vi "DeviceSwitch.vi"(8 "error in (no error)":errorcluster caption="错误输入（无错误）", 9 "Device Index":i32, 10 "Open":bool, 11 "handle":u64) -> (0 "error out":errorcluster caption="错误输出", 2 "function return":i32, 3 "handle out":u64, 5 "Description":string, 7 "SerialNumber":string)   [LabVIEW 2018]
doc: "Set Open True to open device by Device Index or False to close device by handle."
uses:
  InstrumentsPlayground.lvlib
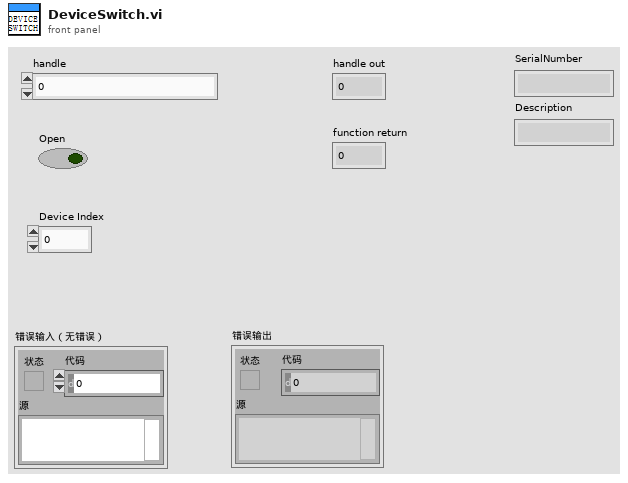
[diagram p1: front panel]
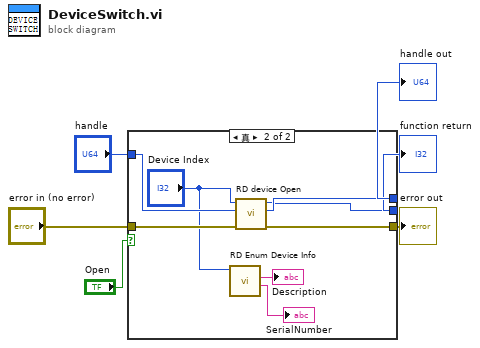
[diagram p0: block diagram]
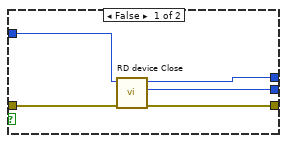
[diagram p2: hidden frame]
diagram:
  n1 = case shown="真" "Open" {
    tunnel: "handle" -> [w11 w18]
    tunnel: [w10 w16] -> w4
    tunnel: [w9 w15] -> w3
    tunnel: [w8 w19] -> w2
    tunnel: "error in (no error)" -> [w7 w17]
    frame False {
      n2 = call "RD device Close.vi"("error in (no error)"=w7, "ftHandle"=w11) -> ("error out"=w8:errorcluster, "function return"=w9:i32, "ftHandle out"=w10:u64)  [unwired: 7 in]
    }
    frame True {
      n3 = call "RD Enum Device Info.vi"("i"="Device Index") -> ("SerialNumber out"=→"SerialNumber":string, "Description out"=→"Description":string)  [unwired: 6 in, 3 out]
      n4 = call "RD device Open.vi"("error in (no error)"=w17, "ftHandle"=w18, "i"="Device Index") -> ("error out"=w19:errorcluster, "ftHandle out"=w16:u64, "function return"=w15:i32)  [unwired: 6 in]
    }
  }
  "error out" <- w2
  "function return" <- w3
  "handle out" <- w4
